vi "240124_Init_Nikon.vi"(8 "error in (no error)":errorcluster) -> (0 "error out":errorcluster, 3 "Nikon cluster":T1)   [LabVIEW 2023]
doc: "This VI initializes the Nikon TI2 microscope"
panel:
  in  "NikonTi2AxLib.INikonTi2AxMicroscope":refnum<k7>
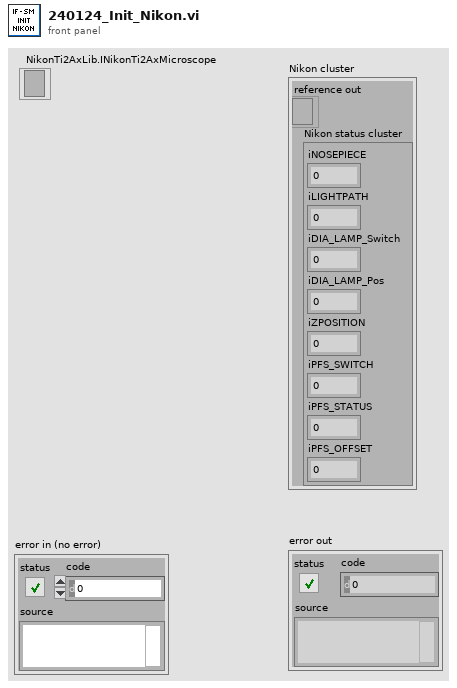
[diagram p1: front panel]
types:
  T1 = cluster{"reference out":refnum<k7>, "Nikon status cluster":cluster{"iNOSEPIECE":i32, "iLIGHTPATH":i32, "iDIA_LAMP_Switch":i32, "iDIA_LAMP_Pos":i32, "iZPOSITION":i32, "iPFS_SWITCH":i32, "iPFS_STATUS":i32, "iPFS_OFFSET":i32}}
  T2 = cluster{"iNOSEPIECE":i32, "iLIGHTPATH":i32, "iDIA_LAMP_Switch":i32, "iDIA_LAMP_Pos":i32, "iZPOSITION":i32, "iPFS_SWITCH":i32, "iPFS_STATUS":i32, "iPFS_OFFSET":i32}
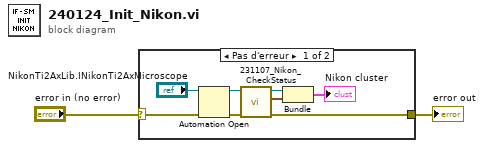
[diagram p0: block diagram]
diagram:
  n1 = case shown="Pas d'erreur" "error in (no error)" {
    selector: "error in (no error)" -> [w9 w11]
    tunnel: [w7 w11] -> w1
    frame No Error {
      n2 = Automation Open(error in (no error)=w9, Automation Refnum="NikonTi2AxLib.INikonTi2AxMicroscope") -> (Automation Refnum=w6:refnum<k7>, error out=w8:errorcluster)  [unwired: 2 in]
      n3 = call "231107_Nikon_CheckStatus.vi"("error in"=w8, "NikonTi2AxLib.INikonTi2AxMicroscope"=w6) -> ("error out"=w7:errorcluster, "Nikon status cluster"=w4:T2, "reference out"=w5:refnum<k7>)  [unwired: 7 in]
      n4 = Bundle("reference out"=w5, "Nikon status cluster"=w4) -> (→"Nikon cluster":T1)  [unwired: 1 in]
    }
    frame Error {
    }
  }
  "error out" <- w1
